vi "002 Comparació aleatoris.vi"() -> ()   [LabVIEW 2019]
panel:
  out "Nombre d'iteracions":dbl
  out "Valor aleatori":dbl
  in  "Entra un nombre":dbl min=0.0 max=10000.0 step=1.0
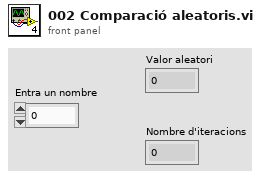
[diagram p1: front panel]
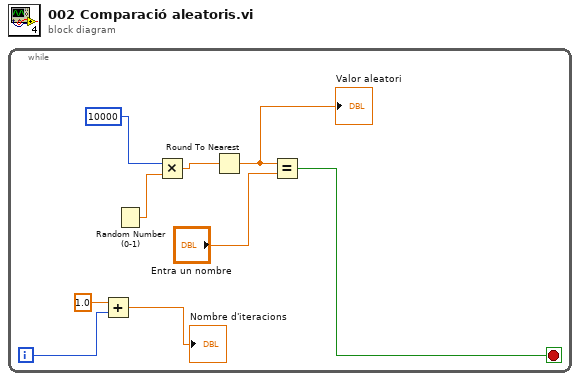
[diagram p0: block diagram]
diagram:
  n1 = while {
    i -> [w3]
    stop <- w8 stop-if-true
    n2 = Add(x=1.0, y=w3) -> (x+y=→"Nombre d'iteracions":dbl)
    n3 = Random Number (0-1)() -> (number: 0 to 1=w9:dbl)
    n4 = Multiply(x=10000, y=w9) -> (x*y=w1:dbl)
    n5 = Round To Nearest(number=w1) -> (nearest integer value=w2:dbl)
    "Valor aleatori" <- w2
    n6 = Equal?(x=w2, y="Entra un nombre") -> (x = y?=w8:bool)
  }
